vi "TCP.IP Client for Ripple Detection_maybe3.vi"() -> ()   [LabVIEW 2021]
doc: "Demonstrates how to open a connection to an TCP server, read the data being sent, and display the data on a chart. This VI is designed to stop if the TCP connection is terminated."
uses:
  <vilib>/Analysis/3filter.llb/Butterworth Filter (DBL).vi
  <vilib>/ptbypt/NI_PtbyPt.lvlib
  <vilib>/Analysis/NI_AALBase.lvlib
panel:
  in  "File Name":path=path "F:/Career/Work/From Now/Book2.csv"
  out "Array Size 3":u32
  out "RMS2>RMS1 for 3 data":dynamicdata(graph)
  out "Array Size":u32
  in  "Boolean":bool
  in  "Server Closed":string="The server VI closed the connection."
  out "Raw Data":dbl[](graph)
  in  "Stop":bool
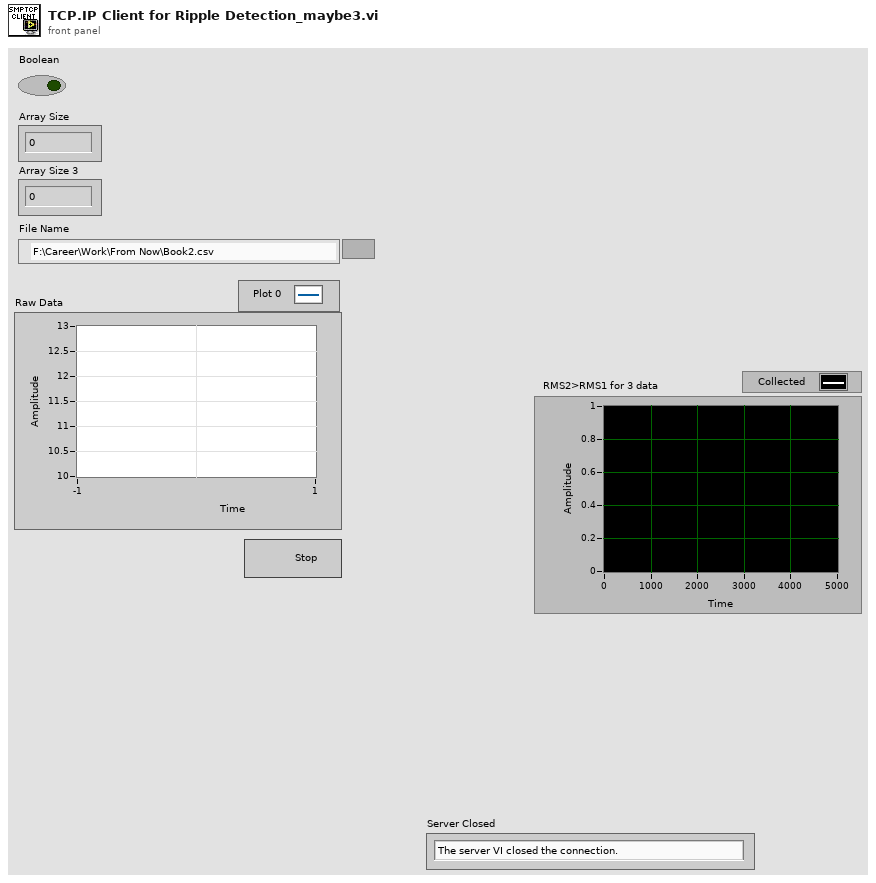
[diagram p1: front panel]
types:
  T1 = enum16{"open", "replace", "create", "open or create", "replace or create", "replace or create with confirmation"}
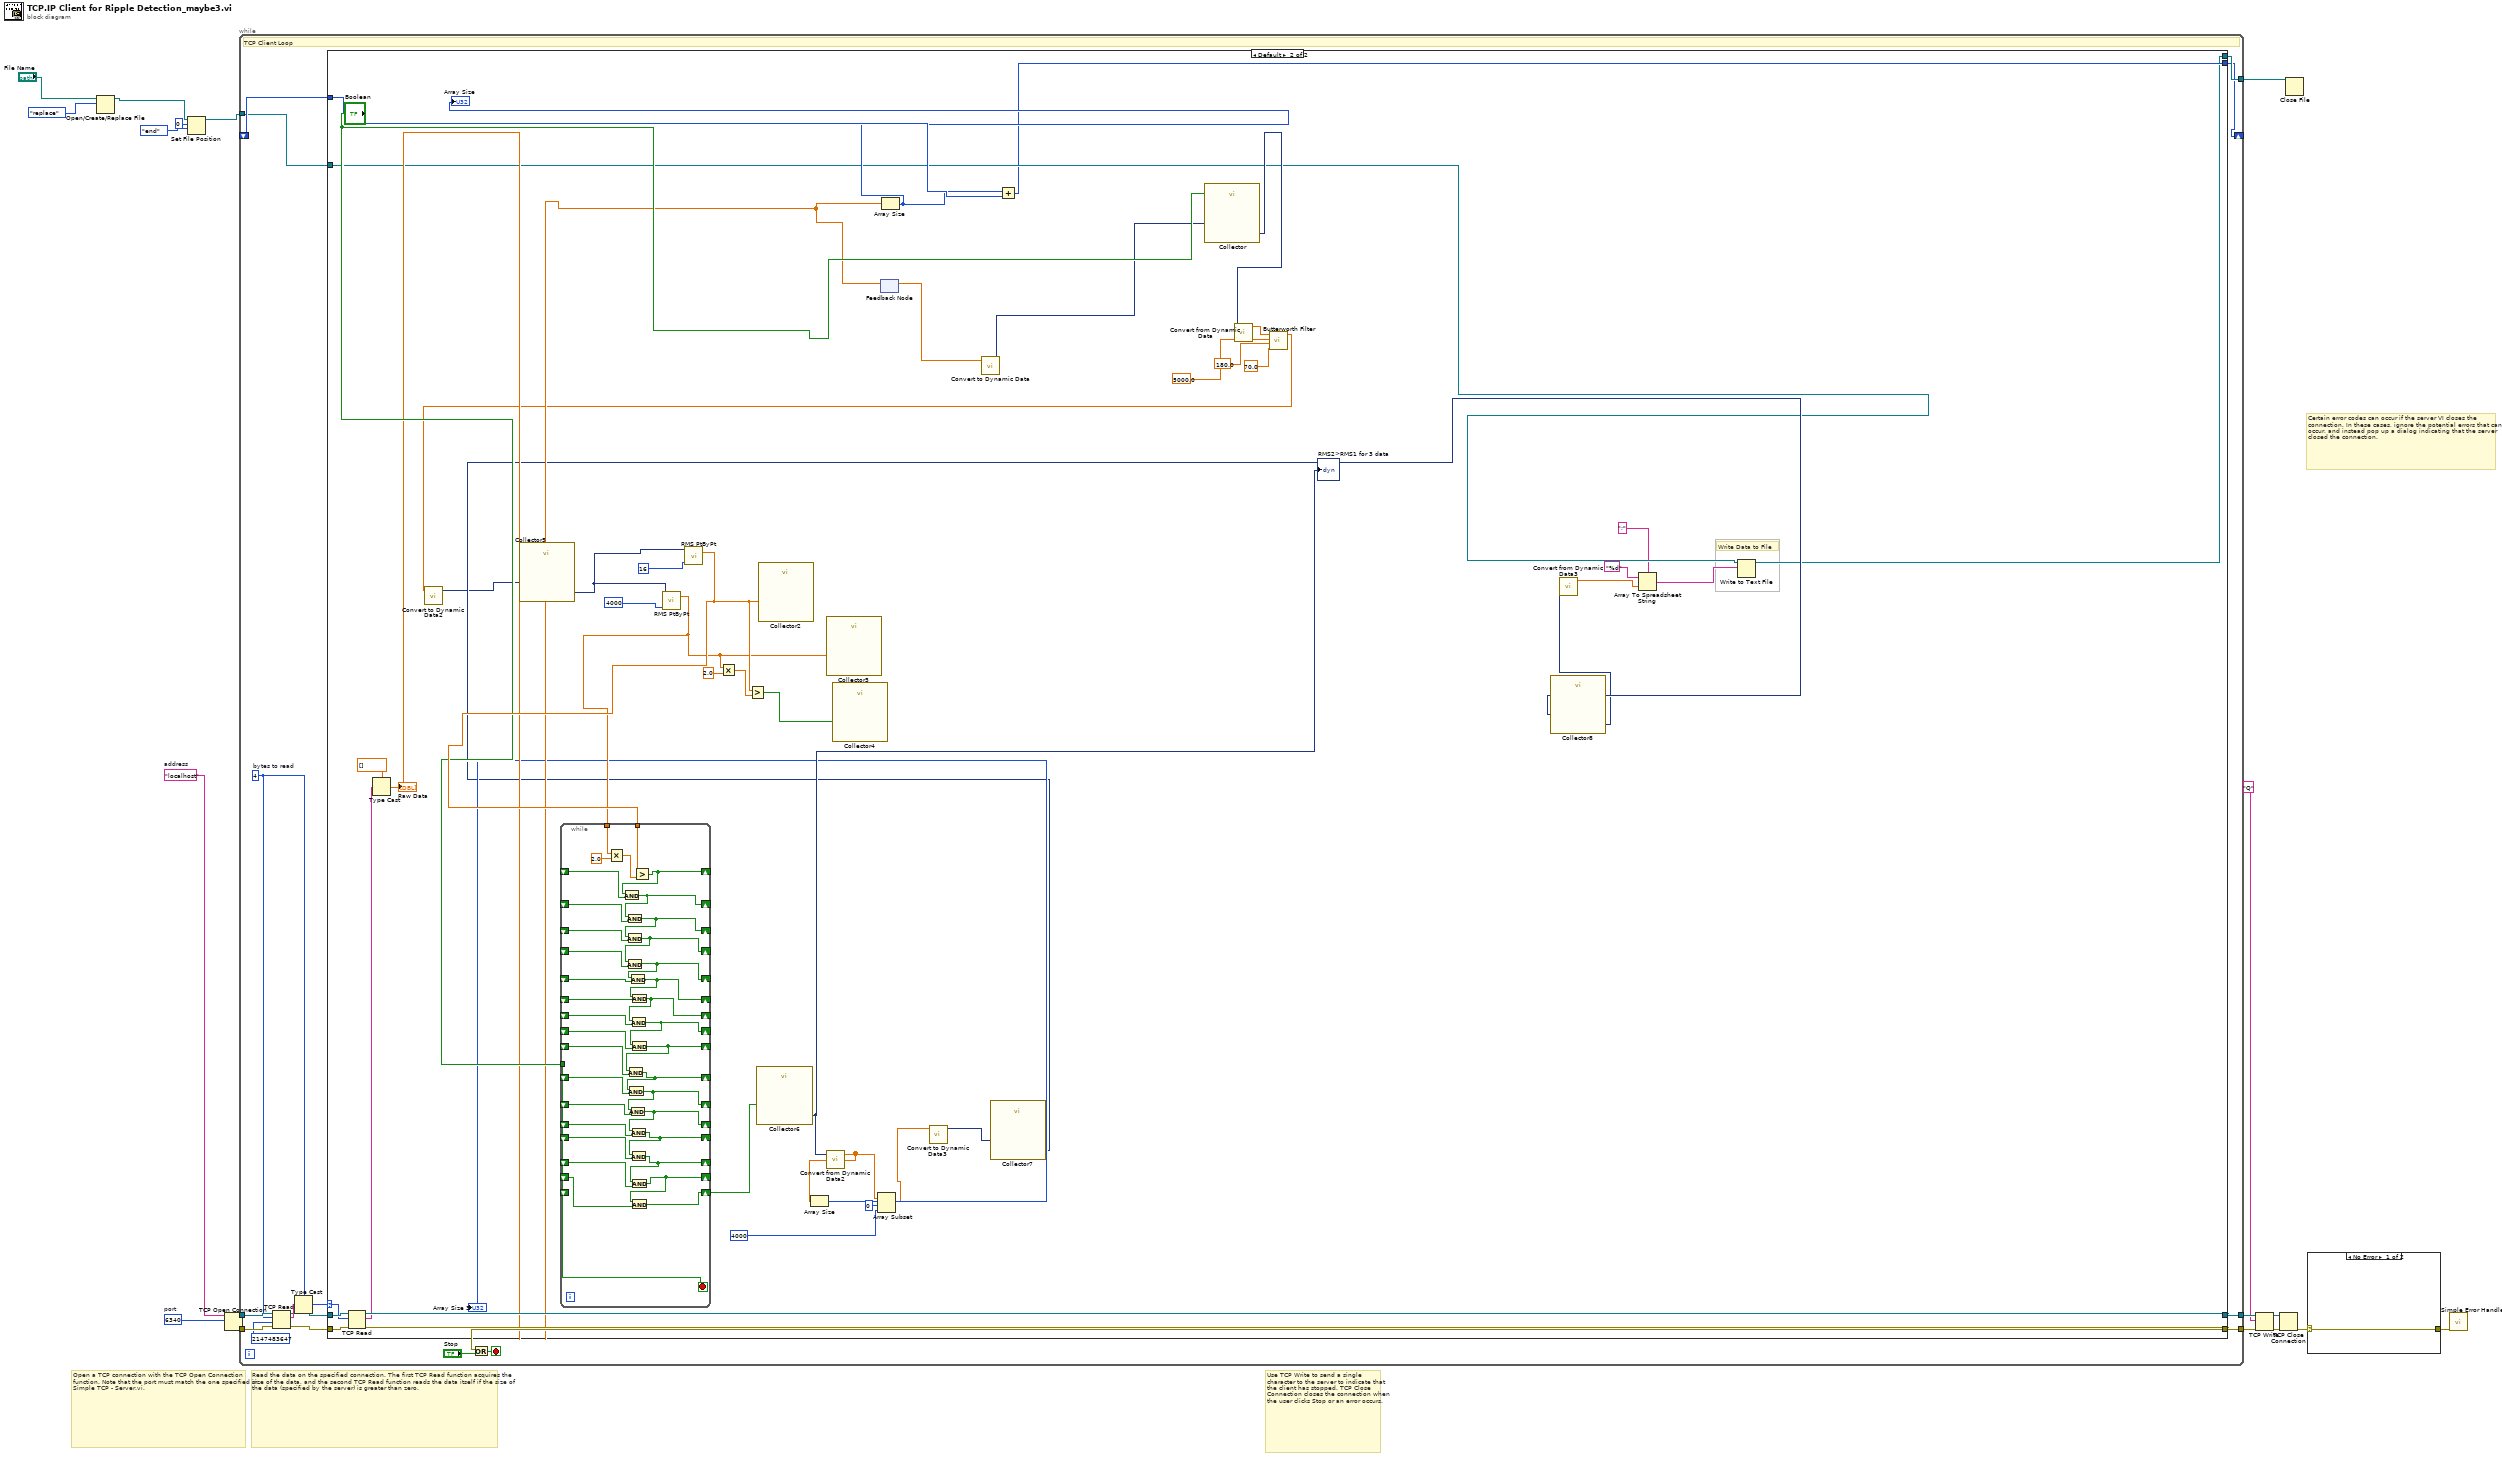
[diagram p0: block diagram]
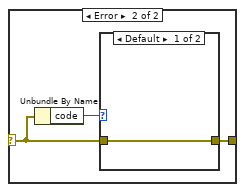
[diagram p2: hidden frame]
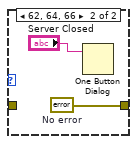
[diagram p3: hidden frame]
diagram:
  w8 = u16 6340  # port
  w9 = "localhost"  # address
  # "Certain error codes can occur if the server VI closes the connection. In these cases, ignore the potential errors that can occur, and instead pop up a dialog indicating that the server closed the connection."
  # "Use TCP Write to send a single character to the server to indicate that the client has stopped. TCP Close Connection closes the connection when the user clicks Stop or an error occurs."
  # "Read the data on the specified connection. The first TCP Read function acquires the size of the data, and the second TCP Read function reads the data itself if the size of the data (specified by the server) is greater than zero."
  # "Open a TCP connection with the TCP Open Connection function. Note that the port must match the one specified in Simple TCP - Server.vi."
  n1 = Open/Create/Replace File(file path (use dialog)="File Name", operation (0:open)=T1."replace") -> (refnum out=w2:refnum<file>)  [unwired: 4 in, 2 out]
  n2 = Set File Position(offset (in bytes) (0)=i64 0, refnum=w2, from (0:start)=enum16{"start", "end", "current"}."end") -> (refnum out=w1:refnum<file>)  [unwired: 1 in, 1 out]
  n3 = TCP Open Connection(address=w9, remote port or service name=w8) -> (connection ID=w18:refnum<k5>, error out=w17:errorcluster)  [unwired: 3 in]
  n4 = while {
    tunnel: w17 -> [w30]
    tunnel: w18 -> [w31]
    tunnel: [w26] -> w15
    tunnel: [w25] -> w13
    shift-right: [w19] -> _
    shift-left: _ -> [w22]
    tunnel: [w20] -> w7
    tunnel: w1 -> [w21]
    stop <- w27 stop-if-true
    w29 = 4  # bytes to read
    # "TCP Client Loop"
    n5 = TCP Read(connection ID=w31, bytes to read=w29, error in (no error)=w30, 9:2147483647 ("timeout ms (25000)")) -> (connection ID out=w33:refnum<k5>, data out=w34:string, error out=w32:errorcluster)  [unwired: 1 in]
    n6 = Type Cast(type=w29, x=w34) -> (*(type *) &x=w24:i32)
    n7 = case shown="Default" w24 {
      selector: w24 -> [_ w77]
      tunnel: w33 -> [w38 w83]
      tunnel: w32 -> [w37 w82]
      tunnel: [w38 w80] -> w26
      tunnel: [w37 w79] -> w25
      tunnel: w22 -> [w36 w72]
      tunnel: [w36 w40] -> w19
      tunnel: w21 -> [w35 w65]
      tunnel: [w35 w39] -> w20
      frame ..0 {
        # "The server has not written any data"
      }
      frame Default {
        # "Write Data to File"
        n8 = TCP Read(connection ID=w83, bytes to read=w77, error in (no error)=w82) -> (connection ID out=w80:refnum<k5>, data out=w78:string, error out=w79:errorcluster)  [unwired: 2 in]
        n9 = Type Cast(type=dbl[] [] ("chart"), x=w78) -> (*(type *) &x=w71:dbl[])
        "Raw Data" <- w71
        n10 = feedback #1() -> (w59:dbl[])  [unwired: 1 in]
        n11 = feedback-in #1(w71) -> ()
        n12 = Array Size(array=w71) -> (size(s)=w70:i32)
        "Array Size" <- w70
        n13 = call "Convert to Dynamic Data"("Array"=w59) -> ("Dynamic Data Type"=w60:dynamicdata)  [unwired: 3 in]
        n14 = Add(x=w70, y=w72) -> (x+y=w40:i32)
        n15 = call "Collector"("Enable"="Boolean", "Signals"=w60) -> ("Collected Signals"=w76:dynamicdata)  [unwired: 8 in, 1 out]
        n16 = call "Convert from Dynamic Data"("Dynamic Data Type"=w76) -> ("Array"=w61:dbl[])  [unwired: 3 in]
        n17 = call-poly <vilib>:"Butterworth Filter.vi"("low cutoff freq: fl"=70.0, "high cutoff freq: fh"=180.0, "sampling freq: fs"=5000.0, "X"=w61) -> ("Filtered X"=w67:dbl[])  [unwired: 4 in, 1 out]
        n18 = call "Convert to Dynamic Data2"("Array"=w67) -> ("Dynamic Data Type"=w53:dynamicdata)  [unwired: 3 in]
        n19 = call "Collector5"("Signals"=w53) -> ("Collected Signals"=w52:dynamicdata)  [unwired: 9 in, 1 out]
        n20 = call <vilib>:"RMS PtByPt.vi"("sample length"=4000, "x"=w52) -> ("rms value"=w74:dbl)  [unwired: 2 in, 1 out]
        n21 = call <vilib>:"RMS PtByPt.vi"("sample length"=16, "x"=w52) -> ("rms value"=w75:dbl)  [unwired: 2 in, 1 out]
        n22 = while {
          tunnel: w75 -> [w117]
          tunnel: w74 -> [w116]
          shift-right: [w111] -> _
          shift-left: _ -> [w112]
          shift-right: [w114] -> _
          shift-left: _ -> [w113]
          tunnel: "Boolean" -> [w115]
          shift-right: [w109] -> _
          shift-left: _ -> [w110]
          shift-right: [w107] -> _
          shift-left: _ -> [w108]
          shift-right: [w106] -> _
          shift-left: _ -> [w105]
          shift-right: [w97] -> _
          shift-left: _ -> [w90]
          shift-right: [w102] -> _
          shift-left: _ -> [w101]
          shift-right: [w104] -> _
          shift-left: _ -> [w103]
          shift-right: [w99] -> _
          shift-left: _ -> [w100]
          shift-right: [w98] -> _
          shift-left: _ -> [w91]
          shift-right: [w96] -> _
          shift-left: _ -> [w89]
          shift-right: [w95] -> _
          shift-left: _ -> [w88]
          shift-right: [w94] -> _
          shift-left: _ -> [w87]
          shift-right: [w93] -> _
          shift-left: _ -> [w86]
          shift-right: [w92] -> _
          shift-left: _ -> [w85]
          shift-right: [w84] -> w46
          shift-left: _ -> [_]
          stop <- w115 stop-if-true
          n23 = Multiply(x=w116, y=2.0) -> (x*y=w118:dbl)
          n24 = Greater?(x=w117, y=w118) -> (0:w114:bool)
          n25 = And(x=w114, y=w113) -> (x .and. y?=w111:bool)
          n26 = And(x=w111, y=w112) -> (x .and. y?=w109:bool)
          n27 = And(x=w109, y=w110) -> (x .and. y?=w107:bool)
          n28 = And(x=w107, y=w108) -> (x .and. y?=w106:bool)
          n29 = And(x=w106, y=w105) -> (x .and. y?=w104:bool)
          n30 = And(x=w104, y=w103) -> (x .and. y?=w102:bool)
          n31 = And(x=w102, y=w101) -> (x .and. y?=w99:bool)
          n32 = And(x=w99, y=w100) -> (x .and. y?=w98:bool)
          n33 = And(x=w98, y=w91) -> (x .and. y?=w97:bool)
          n34 = And(x=w97, y=w90) -> (x .and. y?=w96:bool)
          n35 = And(x=w96, y=w89) -> (x .and. y?=w95:bool)
          n36 = And(x=w95, y=w88) -> (x .and. y?=w94:bool)
          n37 = And(x=w94, y=w87) -> (x .and. y?=w93:bool)
          n38 = And(x=w93, y=w86) -> (x .and. y?=w92:bool)
          n39 = And(x=w92, y=w85) -> (x .and. y?=w84:bool)
        }
        n40 = Multiply(x=w74, y=2.0) -> (x*y=w55:dbl)
        n41 = Greater?(x=w75, y=w55) -> (0:w54:bool)
        n42 = call "Collector6"("Signals"=w46) -> ("Collected Signals"=w69:dynamicdata)  [unwired: 9 in, 1 out]
        "RMS2>RMS1 for 3 data" <- w69
        n43 = call "Collector2"("Signals"=w75) -> ()  [unwired: 9 in, 2 out]
        n44 = call "Collector3"("Signals"=w74) -> ()  [unwired: 9 in, 2 out]
        n45 = call "Convert from Dynamic Data2"("Dynamic Data Type"=w69) -> ("Array"=w48:dbl[])  [unwired: 3 in]
        n46 = Array Size(array=w48) -> (size(s)=→"Array Size 3":i32)
        n47 = call "Collector4"("Signals"=w54) -> ()  [unwired: 9 in, 2 out]
        n48 = Array Subset(array=w48, index=0, length=4000 ("index")) -> (w47:dbl[])
        n49 = call "Convert to Dynamic Data3"("Array"=w47) -> ("Dynamic Data Type"=w51:dynamicdata)  [unwired: 3 in]
        n50 = call "Collector7"("Signals"=w51) -> ("Collected Signals"=w66:dynamicdata)  [unwired: 9 in, 1 out]
        n51 = call "Collector8"("Signals"=w66) -> ("Collected Signals"=w45:dynamicdata)  [unwired: 9 in, 1 out]
        n52 = call "Convert from Dynamic Data3"("Dynamic Data Type"=w45) -> ("Array"=w44:dbl[])  [unwired: 3 in]
        n53 = Array To Spreadsheet String(delimiter (Tab)=";" ("delimiter (\\t)"), array=w44, 3:"%d" ("format string")) -> (spreadsheet string=w43:string)
        n54 = Write to Text File(file (use dialog)=w65, text=w43) -> (refnum out=w39:refnum<file>)  [unwired: 2 in, 2 out]
      }
    }
    n55 = Or(x=w25, y="Stop") -> (x .or. y?=w27:bool)
  }
  n56 = TCP Write(connection ID=w15, data in="Q", error in (no error)=w13) -> (connection ID out=w16:refnum<k5>, error out=w14:errorcluster)  [unwired: 2 out]
  n57 = TCP Close Connection(connection ID=w16, error in (no error)=w14) -> (error out=w11:errorcluster)  [unwired: 1 in, 1 out]
  n58 = Close File(refnum=w7) -> ()  [unwired: 1 in, 2 out]
  n59 = case shown="No Error" w11 {
    selector: w11 -> [w120 w122]
    tunnel: [w120 w121] -> w10
    frame No Error {
    }
    frame Error {
      n60 = Unbundle By Name(w122) -> ("code"=w123:i32)
      n61 = case shown="Default" w123 {
        tunnel: w122 -> [w124 _]
        tunnel: [w124 w126] -> w121
        frame Default {
        }
        frame 62, 64, 66 {
          w126 = errorcluster {"status"=FALSE, "code"=0, "source"=""}  # No error
          n62 = One Button Dialog(message="Server Closed") -> ()  [unwired: 1 in, 1 out]
        }
      }
    }
  }
  n63 = call <vilib>:"Simple Error Handler.vi"("error in (no error)"=w10) -> ()  [unwired: 4 in, 5 out]
